vi "Abre_Certificado_PDF.vi"() -> ()   [LabVIEW 2019]
panel:
  in  "Cancel Button":bool
  out "Horizontal Graduated Bar":u8(slide) scale=0.0..100.0
  in  "TAG":string
  # "CERTIFICADO DE CALIBRA敲O"
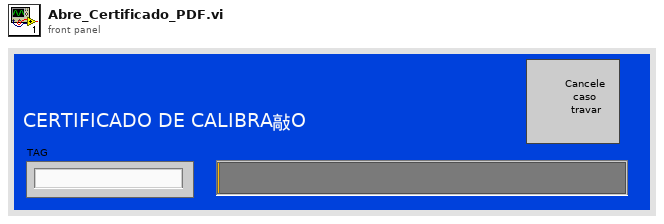
[diagram p1: front panel]
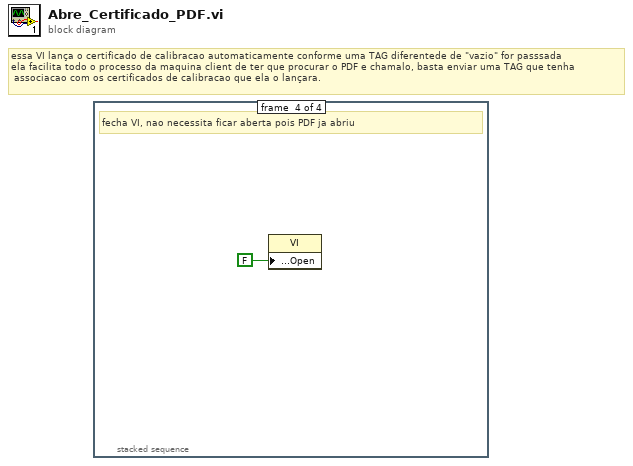
[diagram p0: block diagram]
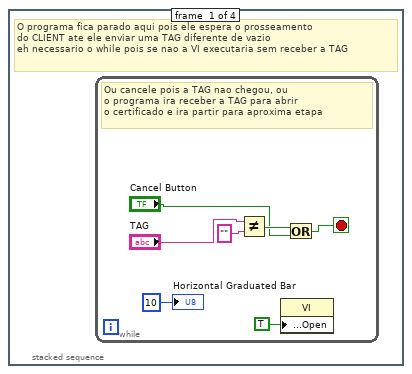
[diagram p2: hidden frame]
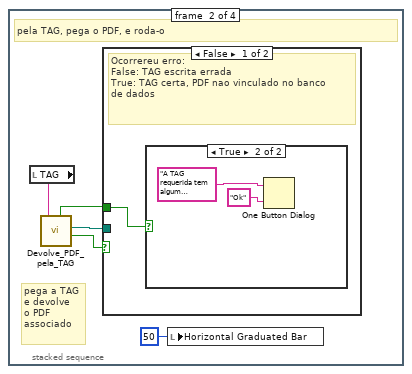
[diagram p3: hidden frame]
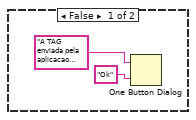
[diagram p4: hidden frame]
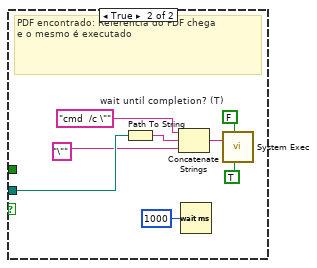
[diagram p5: hidden frame]
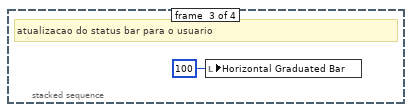
[diagram p6: hidden frame]
diagram:
  # "essa VI lança o certificado de calibracao automaticamente conforme uma TAG diferentede de \"vazio\" for passsada\nela facilita todo o processo da maquina client de ter que procurar o PDF e chamalo, basta enviar uma TAG que tenha\n associacao com os certificados de calibracao que ela o lançara."
  n1 = stacked-sequence {
    frame #0 {
      # "O programa fica parado aqui pois ele espera o prosseamento\ndo CLIENT ate ele enviar uma TAG diferente de vazio\neh necessario o while pois se nao a VI executaria sem receber a TAG"
      n2 = while {
        stop <- w3 stop-if-true
        # "Ou cancele pois a TAG nao chegou, ou \no programa ira receber a TAG para abrir\no certificado e ira partir para aproxima etapa"
        n3 = Not Equal?(x="TAG", y="") -> (x != y?=w2:bool)
        n4 = property class="VI"("Front Panel.Open"=TRUE ("Front Panel Window:Open")) -> ()  [unwired: 2 in, 2 out]
        n5 = Or(x=w2, y="Cancel Button") -> (x .or. y?=w3:bool)
        "Horizontal Graduated Bar" <- u8 10 ("Horizontal Graduated Bar")
      }
    }
    frame #1 {
      # "pega a TAG\ne devolve\no PDF \nassociado"
      # "pela TAG, pega o PDF, e roda-o"
      n6 = local read "TAG"() -> (w12:string)
      n7 = call "Devolve_PDF_pela_TAG.vi"("TAG"=w12) -> ("found?"=w10:bool, "path"=w11:path, "TAG existe?"=w9:bool)  [unwired: 6 in]
      n8 = case shown="False" w10 {
        tunnel: w11 -> [_ w25]
        tunnel: w9 -> [w13 _]
        frame False {
          # "Ocorrereu erro:\nFalse: TAG escrita errada\nTrue: TAG certa, PDF nao vinculado no banco\nde dados"
          n9 = case shown="True" w13 {
            frame False {
              n10 = One Button Dialog(message="A TAG enviada pela aplicacao referente ao instrumento pode estar escrita errada ou mal vinculada, o programa não a encontrou no banco de dados vinculada aos certificados de calibração.\nVerifique na aplicacao se a TAG esta sendo enviada corretamente, olhe exemplos que deram certos.", button name ("OK")="Ok") -> ()  [unwired: 1 out]
            }
            frame True {
              n11 = One Button Dialog(message="A TAG requerida tem algum problema com o Certificado De Calibração\nO problema pode ser a falta de inserção do PDF correto referenciando a devida variável.\nSelecione para editar as relações entre variáveis e PDFs para corrigir o problema!\n", button name ("OK")="Ok") -> ()  [unwired: 1 out]
            }
          }
        }
        frame True {
          w24 = FALSE  # wait until completion? (T)
          # "PDF encontrado: Referencia do PDF chega \ne o mesmo é executado"
          n12 = Path To String(path=w25) -> (string=w20:string)
          n13 = Concatenate Strings("cmd  /c \"", w20, "\"") -> (w22:string)
          n14 = Wait (ms)(milliseconds to wait=u32 1000) -> ()  [unwired: 1 out]
          n15 = call <vilib>:"System Exec.vi"("run minimized? (F)"=TRUE, "wait until completion? (T)"=w24, "command line"=w22) -> ()  [unwired: 5 in, 4 out]
        }
      }
      n16 = local write "Horizontal Graduated Bar"(u8 50 ("Horizontal Graduated Bar")) -> ()
    }
    frame #2 {
      # "atualizacao do status bar para o usuario"
      n17 = local write "Horizontal Graduated Bar"(u8 100 ("Horizontal Graduated Bar")) -> ()
    }
    frame #3 {
      # "fecha VI, nao necessita ficar aberta pois PDF ja abriu"
      n18 = property class="VI"("Front Panel.Open"=FALSE ("Front Panel Window:Open")) -> ()  [unwired: 2 in, 2 out]
    }
  }
